vi "Convert Digital to Analog Waveform.vi"(6 "full scale range":dbl=10.0 format="%#_13g", 7 "channel index":i32, 9 "Number of samples":u32, 10 "Sample rate":dbl, 11 "Digital waveform in":u32[](array[numeric])) -> (1 "codes":u32[](array[numeric]), 2 "Digital waveform out":u32[](array[numeric]), 3 "Waveform":waveform(dbl))   [LabVIEW 2021]
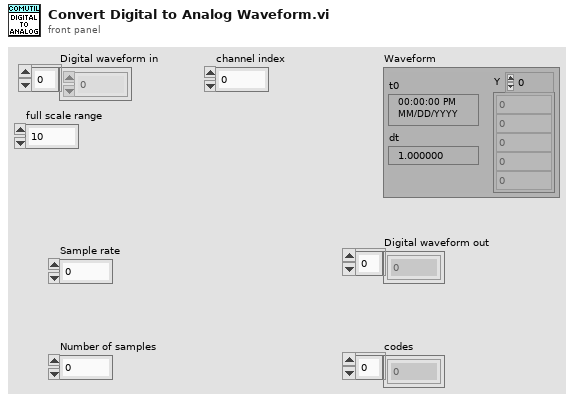
[diagram p1: front panel]
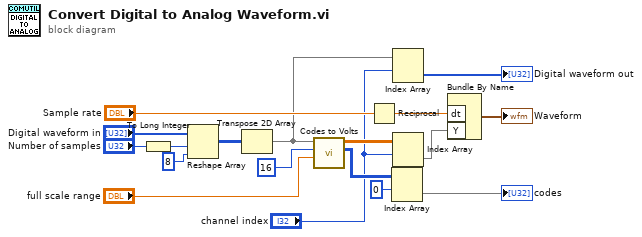
[diagram p0: block diagram]
diagram:
  n1 = To Long Integer(number="Number of samples") -> (32bit integer=w18:i32)
  n2 = Reshape Array("Digital waveform in", w18, 8 ("dimension size")) -> (w10:u32[][])
  n3 = Transpose 2D Array(2D array=w10) -> (transposed array=w3:u32[][])
  n4 = call "Codes to Volts.vi"("full scale range"="full scale range", "number of bits"=16, "data"=w3) -> ("codes"=w6:u32[][], "scaled data"=w13:dbl[][])  [unwired: 7 in]
  n5 = Reciprocal(x="Sample rate") -> (1/x=w14:dbl)
  n6 = Index Array(array=w6, index (row)=0) -> (element=→"codes":u32[])  [unwired: 1 in]
  n7 = Index Array(array=w3, index (row)="channel index") -> (element=→"Digital waveform out":u32[])  [unwired: 1 in]
  n8 = Index Array(array=w13, index (row)="channel index") -> (element=w7:dbl[])  [unwired: 1 in]
  n9 = Bundle By Name("dt"=w14, "Y"=w7) -> (→"Waveform":waveform(dbl))  [unwired: 1 in]
